vi "Read output file string.vi"(8 "error in (no error)":errorcluster, 11 "Shared Memory Configuration in":refnum<class "shared memory configuration.lvclass">) -> (0 "error out":errorcluster, 2 "output file string":string, 3 "Shared Memory Configuration out":refnum<class "shared memory configuration.lvclass">)   [LabVIEW 2013, in "Shared Memory Configuration.lvclass"]
uses:
  shared memory configuration.lvclass
  shared memory configuration.lvclass/shared memory configuration.ctl
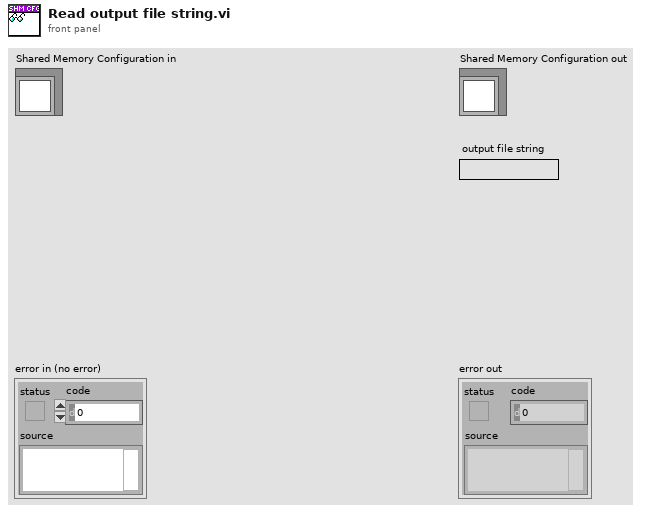
[diagram p1: front panel]
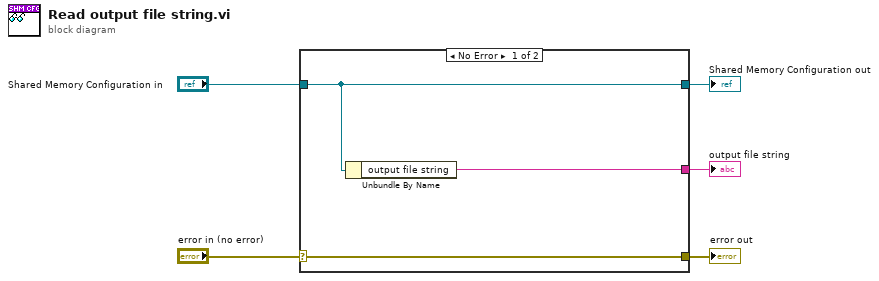
[diagram p0: block diagram]
diagram:
  n1 = case shown="No Error" "error in (no error)" {
    selector: "error in (no error)" -> [w8 w9]
    tunnel: [w8 w9] -> w4
    tunnel: [w7 w10] -> w2
    tunnel: "Shared Memory Configuration in" -> [w7 w10]
    tunnel: [w6 _] -> w1
    frame No Error {
      n2 = Unbundle By Name(w7) -> ("output file string"=w6:string)
    }
    frame Error {
    }
  }
  "error out" <- w4
  "Shared Memory Configuration out" <- w2
  "output file string" <- w1
